vi "Add Service.vi"(6 "Data":string, 7 "safeMode":bool=TRUE, 8 "error in (no error)":errorcluster, 9 "Type Descriptor":string, 10 "Service Name":string, 11 "DIMActor in":refnum<class "DIMActor.lvclass">) -> (0 "error out":errorcluster, 3 "DIMActor out":refnum<class "DIMActor.lvclass">)   [LabVIEW 2012, in "DIMActor.lvlib" / "DIMActor.lvclass"]
doc: "Add a DIM service to publish."
uses:
  DIMActor.lvclass
  DIMActor.lvclass/DIMActor.ctl
  SVN/LV2009/GPL/lib.lib/DimLVEvent/LVDimInterface/LVDimInterface.lvlib
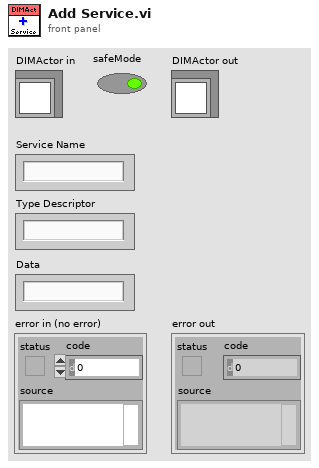
[diagram p1: front panel]
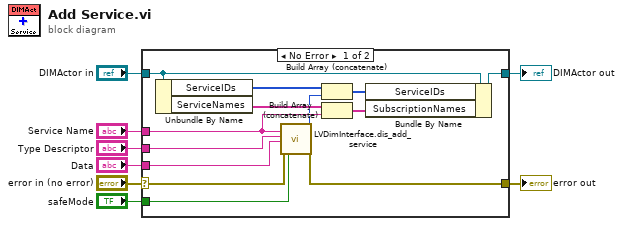
[diagram p0: block diagram]
diagram:
  n1 = case shown="No Error" "error in (no error)" {
    selector: "error in (no error)" -> [w15 w23]
    tunnel: [w10 w23] -> w7
    tunnel: [w18 w22] -> w5
    tunnel: "DIMActor in" -> [w19 w22]
    tunnel: "Service Name" -> [w14 _]
    tunnel: "Type Descriptor" -> [w12 _]
    tunnel: "Data" -> [w11 _]
    tunnel: "safeMode" -> [w9 _]
    frame No Error {
      n2 = Unbundle By Name(w19) -> ("ServiceIDs"=w20:i32[], "ServiceNames"=w17:string[])
      n3 = call "LVDimInterface.dis_add_service.vi"("serviceName"=w14, "typeDescriptor"=w12, "data"=w11, "error in (no error)"=w15, "safeMode"=w9) -> ("my_serviceID"=w13:i32, "error out"=w10:errorcluster)  [unwired: 13 in]
      n4 = Build Array (concatenate)(w20, w13) -> (w21:i32[])
      n5 = Build Array (concatenate)(w17, w14) -> (w16:string[])
      n6 = Bundle By Name(cluster=w19, "ServiceIDs"=w21, "SubscriptionNames"=w16) -> (w18:refnum<class "DIMActor.lvclass">)
    }
    frame Error {
    }
  }
  "error out" <- w7
  "DIMActor out" <- w5
